vi "Sweep Step.vi"(8 "error in (no error)":errorcluster, 11 "Power Supply in":refnum<class "Power Supply.lvclass">) -> (0 "error out":errorcluster, 1 "Done?":bool, 2 "field":dbl[unit], 3 "Power Supply out":refnum<class "Power Supply.lvclass">, 4 "rate":dbl[unit])   [LabVIEW 2023, in "Power Supply.lvclass"]
doc: "As the field sweeps, monitor that the current sweep rate is still appropriate and adjust as necessary."
uses:
  Power Supply.lvclass
  Ramping Mode.ctl
  Power Supply.lvclass/Power Supply.ctl
panel:
  in  "Ramping Mode":T1
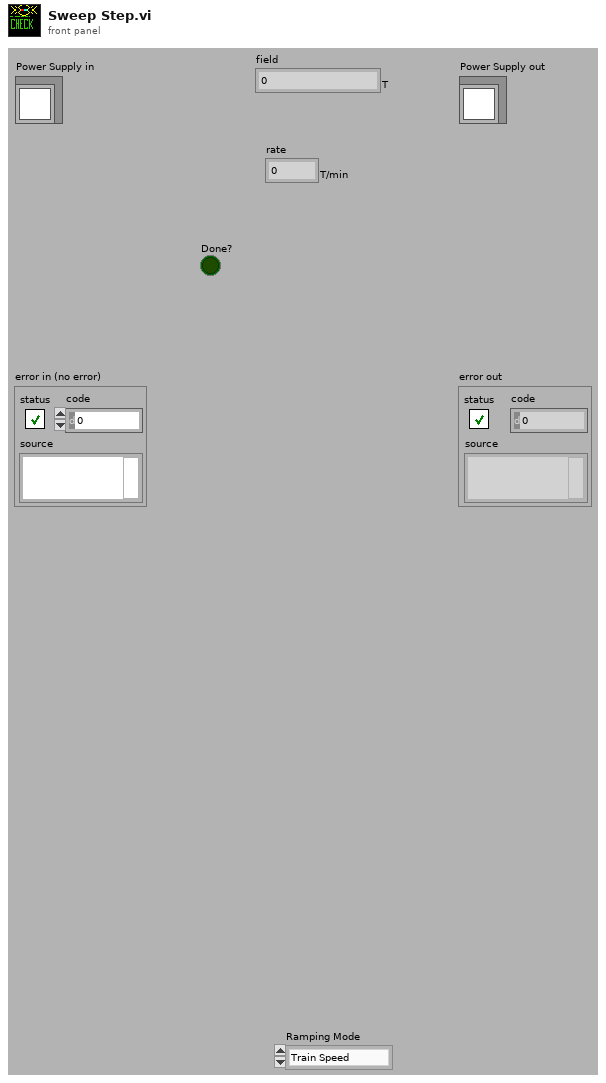
[diagram p1: front panel]
types:
  T1 = typedef "Power Supply.lvclass/Ramping Mode.ctl" = enum16{"Train Speed", "Maximum Speed", "Manual"}
  T2 = typedef "PSIO.ctl" = cluster{"Address":T3, "Version":enum16{"PS", "IPS"}}
  T3 = typedef "OxfordAddress.ctl" = cluster{"Com Port":i32, "ISOBUS Address":i32, "GPIB Address":i16, "Communication":enum16{"RS232", "ISOBUS", "GPIB", "Gateway"}}
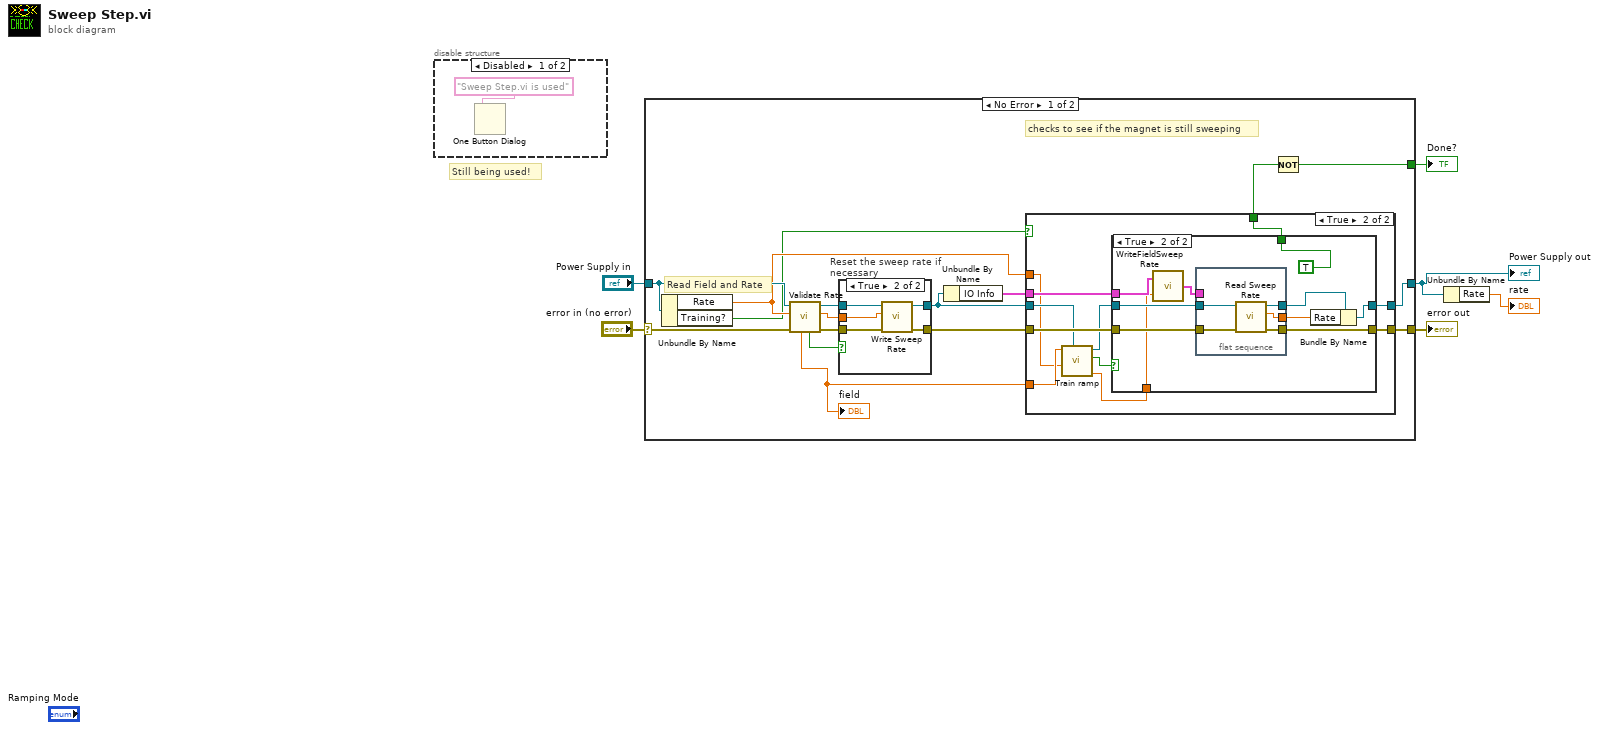
[diagram p0: block diagram]
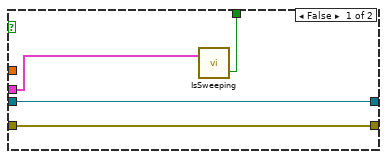
[diagram p3: hidden frame]
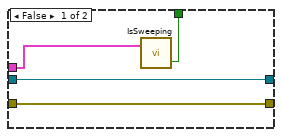
[diagram p4: hidden frame]
diagram:
  # "Still being used!"
  n1 = disable-structure shown="Disabled" {
    frame Disabled {
      n2 = One Button Dialog(message="Sweep Step.vi is used") -> ()  [unwired: 1 in, 1 out]
    }
    frame Enabled {
    }
  }
  n3 = case shown="No Error" "error in (no error)" {
    selector: "error in (no error)" -> [w20 w65]
    tunnel: [w19 _] -> w6
    tunnel: [w17 w65] -> w5
    tunnel: [w13 w66] -> w2
    tunnel: "Power Supply in" -> [w21 w66]
    frame No Error {
      # "checks to see if the magnet is still sweeping"
      # "Read Field and Rate"
      n4 = Unbundle By Name(w21) -> ("Rate"=w10:dbl[unit], "Training?"=w9:bool)
      n5 = call "Validate Rate.vi"("error IO"=w20, "rate"=w10, "Power Supply in"=w21) -> ("error out"=w23:errorcluster, "Coerced rate"=w15:dbl[unit], "Power Supply out"=w22:refnum<class "Power Supply.lvclass">, "Coerced?"=w12:bool, "Field"=w11:dbl[unit])  [unwired: 3 in, 1 out]
      "field" <- w11
      n6 = case "Reset the sweep rate if necessary" shown="True" w12 {
        tunnel: w15 -> [_ w62]
        tunnel: w23 -> [w58 w64]
        tunnel: [w58 w63] -> w18
        tunnel: w22 -> [w59 w61]
        tunnel: [w59 w60] -> w14
        frame False {
        }
        frame True {
          n7 = call-dynamic "Write Sweep Rate.vi"("error in (no error)"=w64, "rate"=w62, "Power Supply in"=w61) -> ("error out"=w63:errorcluster, "Power Supply out"=w60:refnum<class "Power Supply.lvclass">)  [unwired: 7 in]
        }
      }
      n8 = Unbundle By Name(w14) -> ("IO Info"=w16:T2)
      n9 = case shown="True" w9 {
        tunnel: w18 -> [w26 w38]
        tunnel: [w26 w37] -> w17
        tunnel: w16 -> [w25 w35]
        tunnel: w14 -> [w27 w31]
        tunnel: [w27 w36] -> w13
        tunnel: w11 -> [_ w29]
        tunnel: w10 -> [_ w28]
        tunnel: [w24 w34] -> w8
        frame False {
          n10 = call "IsSweeping.vi"("IO Info"=w25) -> ("Sweeping"=w24:bool)  [unwired: 2 out]
        }
        frame True {
          n11 = call "Train ramp.vi"("pwr supply in"=w31, "input"=w28, "field"=w29) -> ("output"=w32:dbl[unit], "change?"=w33:bool, "pwr supply out"=w30:refnum<class "Power Supply.lvclass">)  [unwired: 6 in]
          n12 = case shown="True" w33 {
            tunnel: w38 -> [w41 w50]
            tunnel: [w41 w49] -> w37
            tunnel: w30 -> [w42 w48]
            tunnel: [w42 w47] -> w36
            tunnel: w35 -> [w40 w46]
            tunnel: [w39 TRUE] -> w34
            tunnel: w32 -> [_ w43]
            frame False {
              n13 = call "IsSweeping.vi"("IO Info"=w40) -> ("Sweeping"=w39:bool)  [unwired: 2 out]
            }
            frame True {
              n14 = call "WriteFieldSweepRate.vi"("Sweep rate"=w43, "IO Info"=w46) -> ("IO Info"=w51:T2)
              n15 = flat-sequence {
                tunnel: [w57] -> w45
                tunnel: w48 -> [w56]
                tunnel: [w55] -> w52
                tunnel: w51 -> [_]
                tunnel: w50 -> [w54]
                tunnel: [w53] -> w49
                frame #0 {
                  n16 = call-dynamic "Read Sweep Rate.vi"("error in (no error)"=w54, "Power Supply in"=w56) -> ("error out"=w53:errorcluster, "Field sweep rate"=w57:dbl[unit], "Power Supply out"=w55:refnum<class "Power Supply.lvclass">)  [unwired: 7 in]
                }
              }
              n17 = Bundle By Name(cluster=w52, "Rate"=w45) -> (w47:refnum<class "Power Supply.lvclass">)
            }
          }
        }
      }
      n18 = Not(x=w8) -> (.not. x?=w19:bool)
    }
    frame Error {
    }
  }
  "Done?" <- w6
  "error out" <- w5
  "Power Supply out" <- w2
  n19 = Unbundle By Name(w2) -> ("Rate"=→"rate":dbl[unit])
